vi "create.vi"(0 "HPILCFactory in":refnum<class "HPILCFactory.lvclass">, 5 "HPSettings":T3, 7 "ILCTimings":T2, 9 "HPTimings":T1, 11 "error in (no error)":errorcluster) -> (4 "HPILCFactory out":refnum<class "HPILCFactory.lvclass">, 6 "HPILC":refnum<class "HPILC.lvclass">, 15 "error out":errorcluster)   [LabVIEW 2016, in "RTHPILC.lvlib" / "HPILCFactory.lvclass"]
uses:
  HPILCFactory.lvclass
  DataTypes/HPSettings.ctl
  Common_RT_ILC/DataTypes/ILCSettings.ctl
  HPILC/HPILC.lvclass
  D:/Code/ts_M1M3Support/Common_RT_ILC/ILC/ILC.lvclass
  Common_RT_ILC/DataTypes/ILCTimings.ctl
  DataTypes/HPTimings.ctl
  DataTypes/HPData.ctl
  DataTypes/HPConstants.ctl
  DataTypes/HPCommand.ctl
  DataTypes/HPTelemetry.ctl
  DataTypes/HPResponses.ctl
  Common_RT_Modbus/DataTypes/ExceptionCodes.ctl
  DataTypes/HPTimestamps.ctl
  Common_RT_ILC/ILCFactory/ILCFactory.lvclass
  HPILC/HPILC.lvclass/HPILC.ctl
  Common_RT_Modbus/RTModbus.lvlib
  RTHPILC.lvlib
  Common_RT_ILC/RTILC.lvlib
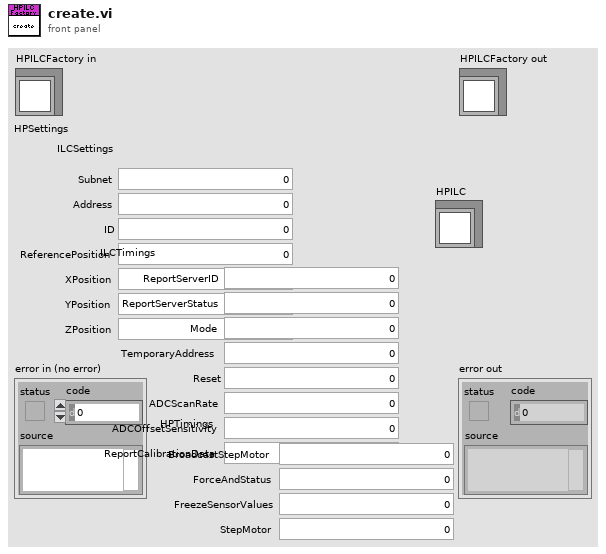
[diagram p1: front panel]
types:
  T1 = typedef "RTHPILC.lvlib/HPTimings.ctl" = cluster{"BroadcastStepMotor":u32, "ForceAndStatus":u32, "FreezeSensorValues":u32, "StepMotor":u32}
  T2 = typedef "RTILC.lvlib/ILCTimings.ctl" = cluster{"ReportServerID":u32, "ReportServerStatus":u32, "Mode":u32, "TemporaryAddress":u32, "Reset":u32, "ADCScanRate":u32, "ADCOffsetSensitivity":u32, "ReportCalibrationData":u32}
  T3 = typedef "RTHPILC.lvlib/HPSettings.ctl" = cluster{"ILCSettings":T4, "ID":i16, "ReferencePosition":i32, "XPosition":sgl, "YPosition":sgl, "ZPosition":sgl}
  T4 = typedef "RTILC.lvlib/ILCSettings.ctl" = cluster{"Subnet":u8, "Address":u8}
  T5 = typedef "RTHPILC.lvlib/HPData.ctl" = cluster{"Constants":T6, "Command":T7, "Telemetry":T8, "Responses":T9, "Timings":T1, "Timestamps":T11}
  T6 = typedef "RTHPILC.lvlib/HPConstants.ctl" = cluster{"ID":i16, "ReferencePosition":i32, "XPosition":sgl, "YPosition":sgl, "ZPosition":sgl}
  T7 = typedef "RTHPILC.lvlib/HPCommand.ctl" = cluster{"Steps":i8}
  T8 = typedef "RTHPILC.lvlib/HPTelemetry.ctl" = cluster{"ILCFault":bool, "LimitSwitchCWOperated":bool, "LimitSwitchCCWOperated":bool, "BroadcastCounter":u8, "SSIEncoderValue":i32, "LoadCellForce":sgl}
  T9 = typedef "RTHPILC.lvlib/HPResponses.ctl" = cluster{"StepMotor":T10, "ForceAndStatus":T10}
  T10 = typedef "RTModbus.lvlib/ExceptionCodes.ctl" = u16
  T11 = typedef "RTHPILC.lvlib/HPTimestamps.ctl" = cluster{"StepMotor":dbl, "ForceAndStatus":dbl}
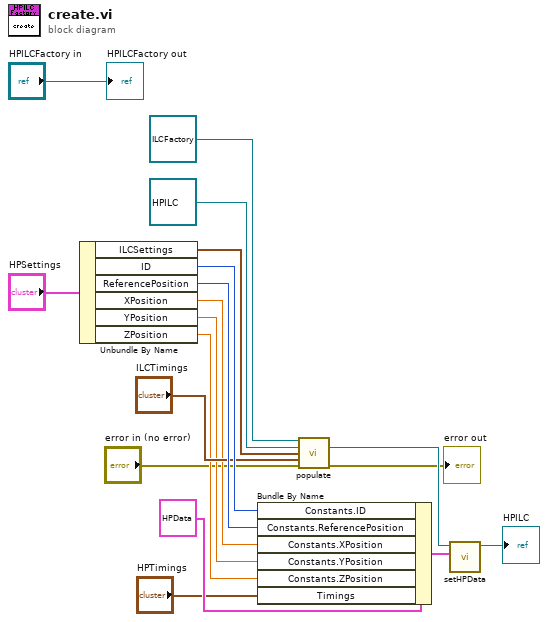
[diagram p0: block diagram]
diagram:
  n1 = Unbundle By Name("HPSettings") -> ("ILCSettings"=w8:T4, "ID"=w13:i16, "ReferencePosition"=w12:i32, "XPosition"=w5:sgl, "YPosition"=w4:sgl, "ZPosition"=w3:sgl)
  n2 = Bundle By Name(cluster=T5 {"Constants"={"ID"=0, "ReferencePosition"=0, "XPosition"=0.0, "YPosition"=0.0, "ZPosition"=0.0}, "Command"={"Steps"=0}, "Telemetry"={"ILCFault"=FALSE, "LimitSwitchCWOperated"=FALSE, "LimitSwitchCCWOperated"=FALSE, "BroadcastCounter"=0, "SSIEncoderValue"=0, "LoadCellForce"=0.0}, "Responses"={"StepMotor"=0, "ForceAndStatus"=0}, "Timings"={"BroadcastStepMotor"=0, "ForceAndStatus"=0, "FreezeSensorValues"=0, "StepMotor"=0}, "Timestamps"={"StepMotor"=0.0, "ForceAndStatus"=0.0}} ("HPData"), "Constants.ID"=w13, "Constants.ReferencePosition"=w12, "Constants.XPosition"=w5, "Constants.YPosition"=w4, "Constants.ZPosition"=w3, "Timings"="HPTimings") -> (w15:T5)
  n3 = call "populate.vi"("ILCFactory in"=refnum<class "ILCFactory.lvclass"> refnum ("RTILC.lvlib:ILCFactory.lvclass"), "ILC in"=refnum<class "HPILC.lvclass"> refnum ("RTHPILC.lvlib:HardPointActuator.lvclass"), "Settings"=w8, "Timings"="ILCTimings", "error in (no error)"="error in (no error)") -> ("ILC out"=w9:refnum<class "HPILC.lvclass">, "error out"=→"error out":errorcluster)  [unwired: 8 in, 1 out]
  n4 = call "setHPData.vi"("HPData"=w15, "HPILC in"=w9) -> ("HPILC out"=→"HPILC":refnum<class "HPILC.lvclass">)  [unwired: 9 in]
  "HPILCFactory out" <- "HPILCFactory in"
